vi "Page_Windows_Security_Write.vi"(6 "ctlReferences":T1, 8 "error in (no error)":errorcluster, 11 "IB_MSI in":refnum<class "IB_MSI.lvclass">) -> (0 "error out":errorcluster, 3 "IB_MSI out":refnum<class "IB_MSI.lvclass">)   [LabVIEW 2020, in "IB_MSI.lvclass"]
uses:
  <vilib>/AppBuilder/IB_Classes/MSI/IB_MSI.lvclass
  <vilib>/AppBuilder/IB_Classes/MSI/IB_MSI.lvclass/IB_MSI.ctl
  <resource>/Framework/Providers/Common/provcom_StringGlobals.vi
  <resource>/Framework/Providers/Builds/AppBuilder/AB_UI_Page_Windows_Security_References.ctl
  <resource>/Framework/Providers/Common/provcom_BrowseProjectFile.ctl
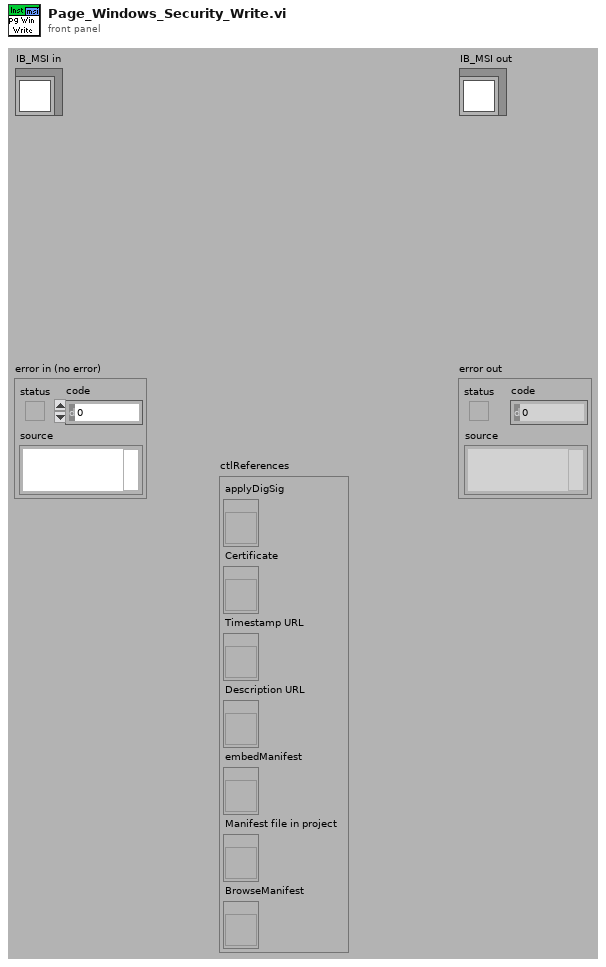
[diagram p1: front panel]
types:
  T1 = typedef "AB_UI_Page_Windows_Security_References.ctl" = cluster{"applyDigSig":refnum<vi>, "Certificate":refnum<vi>, "Timestamp URL":refnum<vi>, "Description URL":refnum<vi>, "embedManifest":refnum<vi>, "Manifest file in project":refnum<vi>, "BrowseManifest":refnum<vi>}
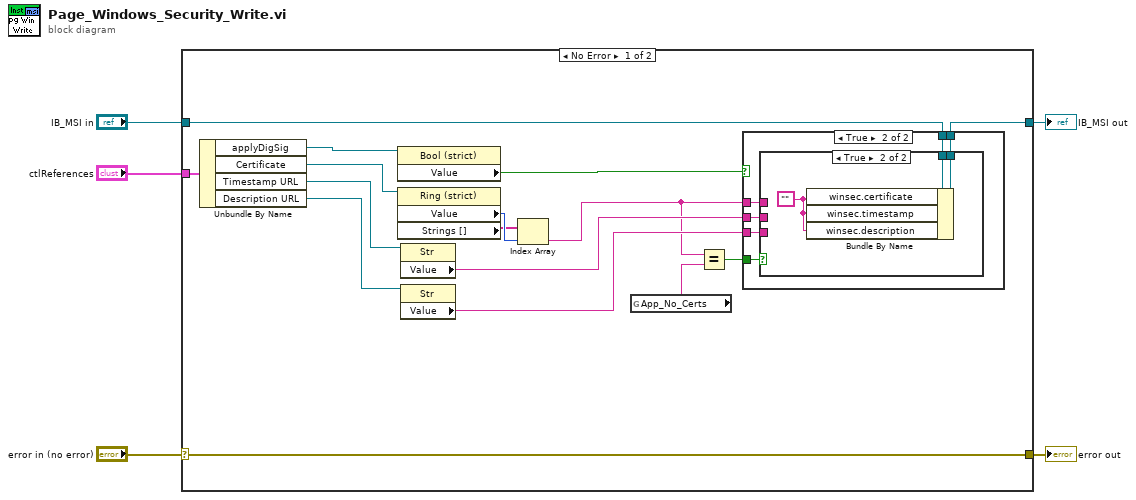
[diagram p0: block diagram]
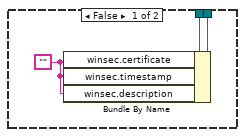
[diagram p2: hidden frame]
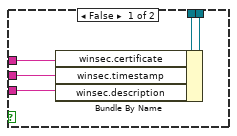
[diagram p3: hidden frame]
diagram:
  n1 = case shown="No Error" "error in (no error)" {
    selector: "error in (no error)" -> [w21 w40]
    tunnel: [w21 w40] -> w3
    tunnel: "ctlReferences" -> [w20 _]
    tunnel: [w9 w39] -> w4
    tunnel: "IB_MSI in" -> [w19 w39]
    frame No Error {
      n2 = Unbundle By Name(w20) -> ("applyDigSig"=w18:refnum<vi>, "Certificate"=w16:refnum<vi>, "Timestamp URL"=w13:refnum<vi>, "Description URL"=w11:refnum<vi>)
      n3 = property class="Bool (strict)"(reference=w18) -> ("Value"=w17:bool)  [unwired: 1 in, 2 out]
      n4 = property class="Ring (strict)"(reference=w16) -> ("Value"=w15:u16, "Strings []"=w14:string[])  [unwired: 1 in, 2 out]
      n5 = property class="Str"(reference=w13) -> ("Value"=w12:string)  [unwired: 1 in, 2 out]
      n6 = property class="Str"(reference=w11) -> ("Value"=w10:string)  [unwired: 1 in, 2 out]
      n7 = Index Array(array=w14, index=w15) -> (element=w7:string)
      n8 = global read "provcom_StringGlobals.vi" "App_No_Certs"() -> (w8:string)
      n9 = Equal?(x=w7, y=w8) -> (x = y?=w6:bool)
      n10 = case shown="True" w17 {
        tunnel: w19 -> [w23 w30]
        tunnel: [w22 w29] -> w9
        tunnel: w7 -> [_ w28]
        tunnel: w12 -> [_ w27]
        tunnel: w10 -> [_ w26]
        tunnel: w6 -> [_ w25]
        frame False {
          w24 = ""
          n11 = Bundle By Name(cluster=w23, "winsec.certificate"=w24, "winsec.timestamp"=w24, "winsec.description"=w24) -> (w22:refnum<class "IB_MSI.lvclass">)
        }
        frame True {
          n12 = case shown="True" w25 {
            tunnel: w30 -> [w35 w37]
            tunnel: [w34 w36] -> w29
            tunnel: w28 -> [w33 _]
            tunnel: w27 -> [w32 _]
            tunnel: w26 -> [w31 _]
            frame False {
              n13 = Bundle By Name(cluster=w35, "winsec.certificate"=w33, "winsec.timestamp"=w32, "winsec.description"=w31) -> (w34:refnum<class "IB_MSI.lvclass">)
            }
            frame True {
              w38 = ""
              n14 = Bundle By Name(cluster=w37, "winsec.certificate"=w38, "winsec.timestamp"=w38, "winsec.description"=w38) -> (w36:refnum<class "IB_MSI.lvclass">)
            }
          }
        }
      }
    }
    frame Error {
    }
  }
  "error out" <- w3
  "IB_MSI out" <- w4
